vi "Gyro Acc Dec Fwd C2Stop.vi"(4 "Refl. color":sgl=12.0, 6 "Ini. Degrees":sgl, 7 "Threshold to C2":i32=900, 8 "Threshold to De-acc":i32=700, 9 "De-acc":i32=10, 10 "Acc":i32=80, 11 "EV3 in":T1) -> (3 "EV3 out":T1)   [LabVIEW 2016]
uses:
  <vilib>/NXT/Subs/LVHSConnector.ctl
  <vilib>/NXT/LegoClasses/BrickReference/BrickReference.lvclass
  <vilib>/NXT/Block Support/NXT_InputPort.ctl
  <vilib>/NXT/Block Support/NXT_OutputPort.ctl
  <vilib>/NXT/NXTIO Xnodes/NXTIONodeSubVIs/LEGOResetMotors.vi
  <vilib>/NXT/Dual Mode Library/Motors/Rotation.vi
  <vilib>/NXT/Dual Mode Library/Sensors/EV3_Gyro_Angle.vi
  <vilib>/NXT/Dual Mode Library/Sensors/EV3_Color_Reflect.vi
  <vilib>/NXT/NXTIO Xnodes/NXTIONodeSubVIs/NXTMotorSteeringOn.vi
  <vilib>/NXT/NXTIO Xnodes/NXTIONodeSubVIs/NXTStopMotors.vi
  <vilib>/NXT/NXTIO Xnodes/NXTIOXNode/NXTIO.xnode
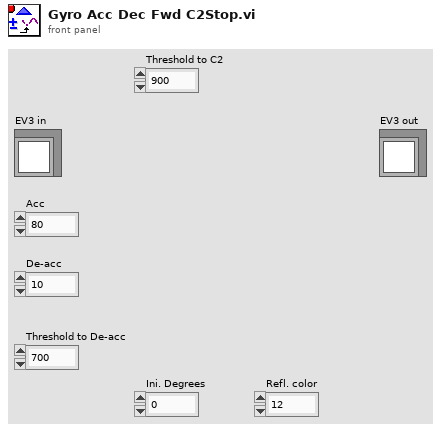
[diagram p1: front panel]
types:
  T1 = typedef "LVHSConnector.ctl" = refnum<class "BrickReference.lvclass">
  T2 = typedef "NXT_OutputPort.ctl" = u8
  T3 = typedef "NXT_InputPort.ctl" = u32
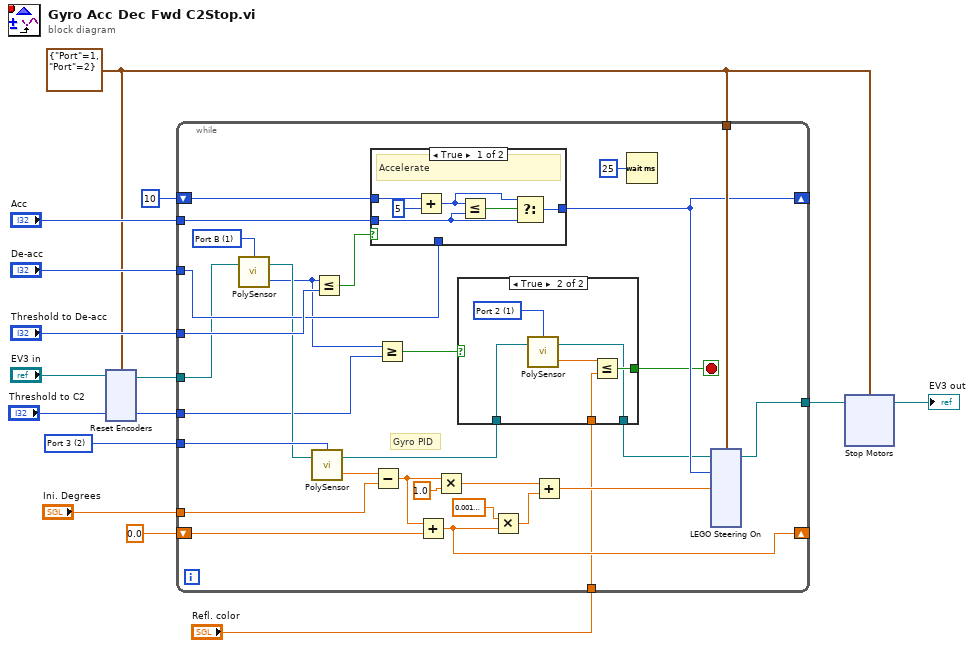
[diagram p0: block diagram]
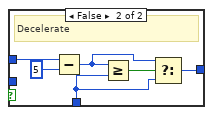
[diagram p3: hidden frame]
diagram:
  w3 = cluster{"Port":T2, "Port":T2} {"Port"=1, "Port"=2} ("Motor")
  w12 = T3 2 items=["Port 1", "Port 2", "Port 3", "Port 4"] ("Port (Gyro)")
  n1 = xnode "Reset Encoders"("Motors"=w3, "NXT/EV3"="EV3 in") -> ("NXT/EV3"=w9:T1)
  n2 = while {
    tunnel: w9 -> [w25]
    tunnel: w12 -> [w33]
    shift-right: [w41] -> _
    shift-left: sgl 0.0 -> [w42]
    tunnel: "Ini. Degrees" -> [w37]
    tunnel: [w32] -> w5
    tunnel: w3 -> [w35]
    shift-right: [w22] -> _
    shift-left: 10 -> [w29]
    tunnel: "De-acc" -> [w26]
    tunnel: "Acc" -> [w28]
    tunnel: "Threshold to De-acc" -> [w27]
    tunnel: "Threshold to C2" -> [w20]
    tunnel: "Refl. color" -> [w15]
    stop <- w18 stop-if-true
    w34 = T2 1 items=["Port A", "Port B", "Port C", "Port D"] ("Port (Port A)")
    # "Gyro PID"
    n3 = call-poly <vilib>:"PolySensor.vi"("NXT/EV3"=w25, "Port (Port A)"=w34) -> ("Angle of Rotation"=w21:i32, "NXT/EV3"=w24:T1)  [unwired: 1 in]
    n4 = call-poly <vilib>:"PolySensor.vi"("NXT/EV3"=w24, "Port (Port 1)"=w33) -> ("Degrees"=w44:sgl, "NXT/EV3"=w17:T1)  [unwired: 1 in]
    n5 = Less Or Equal?(x=w21, y=w27) -> (x <= y?=w23:bool)
    n6 = case shown="True" w23 {
      tunnel: w28 -> [w53 _]
      tunnel: w29 -> [w56 w62]
      tunnel: [w52 w59] -> w22
      tunnel: w26 -> [_ w58]
      frame True {
        # "Accelerate"
        n7 = Add(x=w56, y=5) -> (x+y=w54:i32)
        n8 = Less Or Equal?(x=w54, y=w53) -> (x <= y?=w55:bool)
        n9 = Select(t=w54, s=w55, f=w53) -> (s? t:f=w52:i32)
      }
      frame False {
        # "Decelerate"
        n10 = Subtract(x=w62, y=5) -> (x-y=w60:i32)
        n11 = Greater Or Equal?(x=w60, y=w58) -> (x >= y?=w61:bool)
        n12 = Select(t=w60, s=w61, f=w58) -> (s? t:f=w59:i32)
      }
    }
    n13 = Subtract(x=w44, y=w37) -> (x-y=w36:sgl)
    n14 = Greater Or Equal?(x=w21, y=w20) -> (x >= y?=w19:bool)
    n15 = Add(x=w36, y=w42) -> (x+y=w41:sgl)
    n16 = Multiply(x=w36, y=sgl 1.0 ("K_p")) -> (x*y=w39:sgl)
    n17 = case shown="True" w19 {
      tunnel: [_ w49] -> w18
      tunnel: w17 -> [w45 w48]
      tunnel: [w45 w47] -> w16
      tunnel: w15 -> [_ w46]
      frame False {
      }
      frame True {
        w51 = T3 1 items=["Port 1", "Port 2", "Port 3", "Port 4"] ("Port (Port 1)")
        n18 = call-poly <vilib>:"PolySensor.vi"("NXT/EV3"=w48, "Port (Port 1)"=w51) -> ("Scaled Value"=w50:sgl, "NXT/EV3"=w47:T1)  [unwired: 1 in]
        n19 = Less Or Equal?(x=w50, y=w46) -> (x <= y?=w49:bool)
      }
    }
    n20 = Multiply(x=sgl 0.001 ("K_i"), y=w41) -> (x*y=w38:sgl)
    n21 = Add(x=w39, y=w38) -> (x+y=w30:sgl)
    n22 = Wait (ms)(milliseconds to wait=u32 25) -> ()  [unwired: 1 out]
    n23 = xnode "LEGO Steering On"("Steering 1"=w30, "Power 1"=w22, "Motors"=w35, "NXT/EV3"=w16) -> ("NXT/EV3"=w32:T1)
  }
  n24 = xnode "Stop Motors"("Motors"=w3, "NXT/EV3"=w5) -> ("NXT/EV3"=→"EV3 out":T1)
